vi "DigSeqLogic_On_Delay.vi"(8 "Time":dbl=-1.0, 9 "Delay":dbl=1.0, 11 "Input":bool) -> (1 "Remain":dbl, 3 "Output":bool)   [LabVIEW 2019, in "Trajectory_Library.lvlib"]
doc: "This VI implements a digital \"on delay\". When input is zero, output is zero. When output is true, input goes true after the designated time delay. Once the delay counter has started, the time delay value cannot be changed.\n\nInputs:\n - Input -- Boolean input value\n - Delay -- On delay time in seconds.\n - Time -- Continously counting system time, Seconds. If not wired the FPGA time will be used.\n\nOutputs:\n - Output -- Boolean output value with the on delay applied\n - Remain -- Time remaining for this value to be off in, seconds. Value will be 0 to Delay input value."
uses:
  Trajectory_Library.lvlib
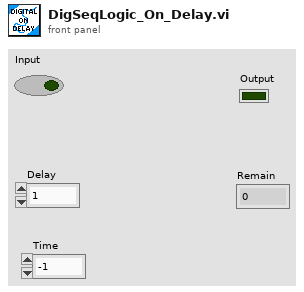
[diagram p1: front panel]
types:
  T1 = typedef "WPILib_Math.lvlib/TIMER.ctl" = cluster{"StartTime":dbl, "Accumulated TIme":dbl, "Running":bool, "semaphore":T2}
  T2 = typedef "Semaphore RefNum" = refnum<k1>
  T3 = typedef "Trajectory_Library.lvlib/TIMER.ctl" = cluster{"StartTime":dbl, "Accumulated TIme":dbl, "Running":bool, "semaphore":T2}
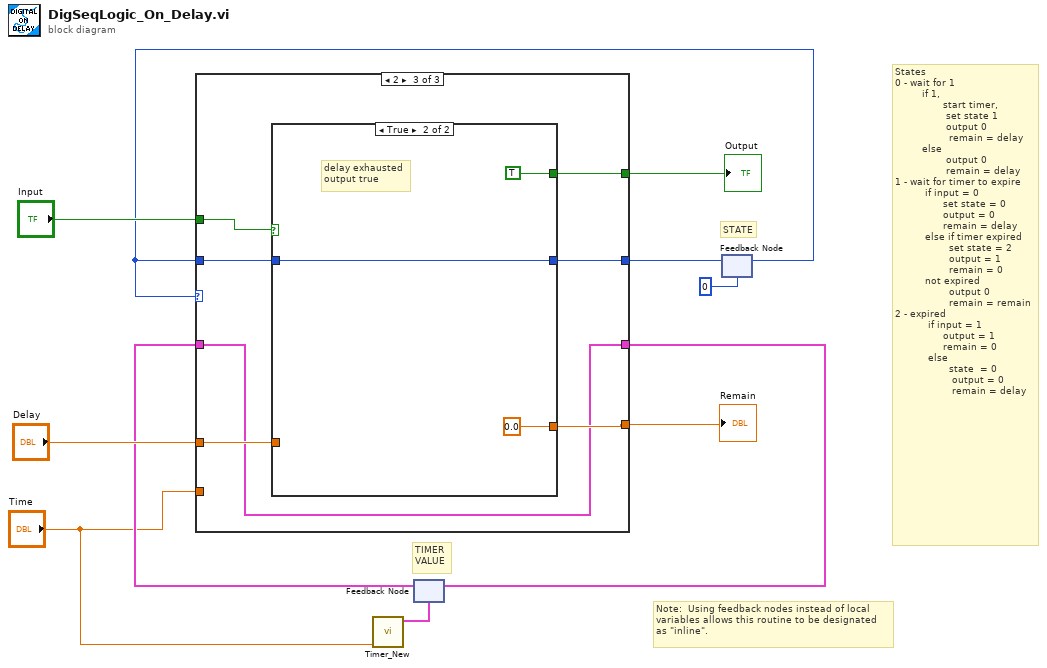
[diagram p0: block diagram]
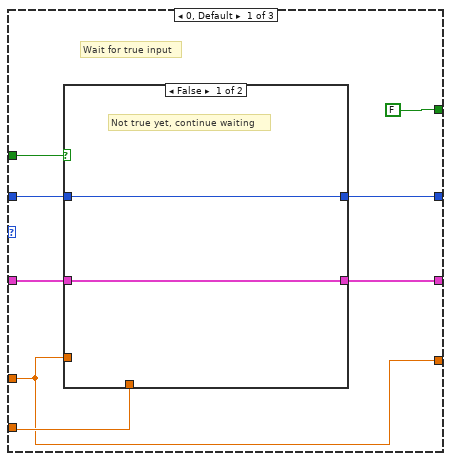
[diagram p2: hidden frame]
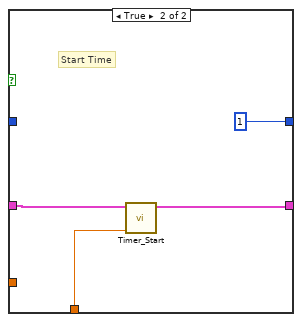
[diagram p3: hidden frame]
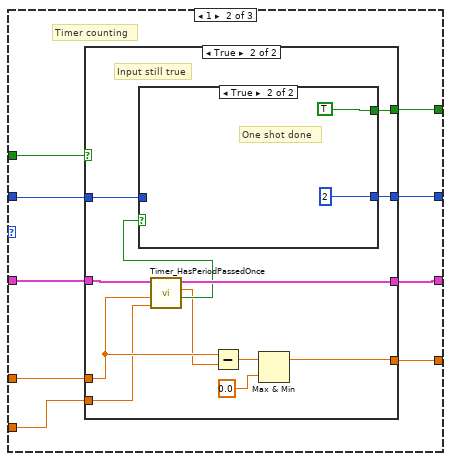
[diagram p4: hidden frame]
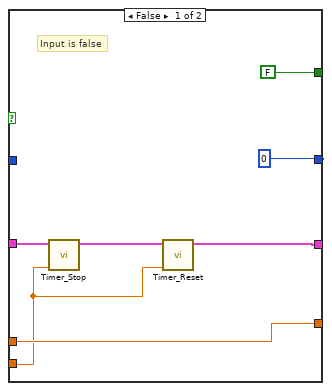
[diagram p5: hidden frame]
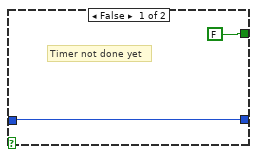
[diagram p6: hidden frame]
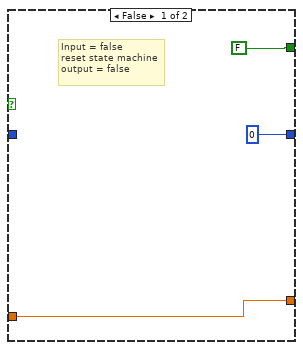
[diagram p7: hidden frame]
diagram:
  # "Note:  Using feedback nodes instead of local\nvariables allows this routine to be designated\nas \"inline\"."
  # "TIMER\nVALUE"
  # "STATE"
  # "States \n0 - wait for 1\n         if 1, \n                start timer, \n                 set state 1\n                 output 0\n                  remain = delay\n         else\n                 output 0\n                 remain = delay    \n1 - wait for timer to expire\n          if input = 0\n                set state = 0\n                output = 0\n                remain = delay\n          else if timer expired\n                  set state = 2\n                  output = 1\n                  remain = 0 \n          not expired\n                  output 0\n                  remain = remain\n2 - expired\n           if input = 1\n                output = 1\n                remain = 0\n           else\n                  state  = 0\n                   output = 0\n                   remain = delay"
  n1 = call "Timer_New.vi"("Pass_Through_Time"="Time") -> ("TIMER"=w4:T1)  [unwired: 10 in]
  n2 = feedback #1(w4) -> (w3:T3)
  n3 = feedback #2(0 ("State")) -> (w6:i32)
  n4 = case shown="2" w6 {
    tunnel: "Delay" -> [w16 w32 w62]
    tunnel: "Time" -> [w19 w30 _]
    tunnel: [FALSE ("Output") w34 w63] -> w10
    tunnel: [w16 w31 w61] -> w9
    tunnel: "Input" -> [w18 w33 w64]
    tunnel: [w15 w29 w60] -> w7
    tunnel: w6 -> [w14 w28 w59]
    tunnel: [w13 w26 w58] -> w2
    tunnel: w3 -> [w12 w27 w58]
    frame 0, Default {
      # "Wait for true input"
      n5 = case shown="False" w18 {
        tunnel: w19 -> [_ w22]
        tunnel: w16 -> [_ _]
        tunnel: [w21 1 ("State")] -> w15
        tunnel: w14 -> [w21 _]
        tunnel: [w20 w23] -> w13
        tunnel: w12 -> [w20 w24]
        frame False {
          # "Not true yet, continue waiting"
        }
        frame True {
          # "Start Time"
          n6 = call "Timer_Start.vi"("Pass_Through_Time"=w22, "in Timer"=w24) -> ("out Timer"=w23:T1)  [unwired: 9 in]
        }
      }
    }
    frame 1 {
      # "Timer counting"
      n7 = case shown="True" w33 {
        tunnel: [FALSE w53] -> w34
        tunnel: [w40 w43] -> w31
        tunnel: w32 -> [w40 w45]
        tunnel: w30 -> [w35 w42]
        tunnel: [0 ("State") w52] -> w29
        tunnel: w28 -> [_ w51]
        tunnel: w27 -> [w38 w50]
        tunnel: [w36 w49] -> w26
        frame False {
          # "Input is false"
          n8 = call "Timer_Stop.vi"("Pass_Through_Time"=w35, "in Timer"=w38) -> ("out Timer"=w37:T3)  [unwired: 9 in]
          n9 = call "Timer_Reset.vi"("Pass_Through_Time"=w35, "in TIMER"=w37) -> ("out TIMER"=w36:T3)  [unwired: 9 in]
        }
        frame True {
          # "Input still true"
          n10 = call "Timer_HasPeriodPassedOnce.vi"("Pass_Through_Time"=w42, "Period"=w45, "in Timer"=w50) -> ("Expired"=w48:bool, "CurrentTImer"=w44:dbl, "out Timer"=w49:T3)  [unwired: 6 in]
          n11 = case shown="True" w48 {
            tunnel: [FALSE TRUE] -> w53
            tunnel: [w54 2 ("State")] -> w52
            tunnel: w51 -> [w54 _]
            frame False {
              # "Timer not done yet"
            }
            frame True {
              # "One shot done"
            }
          }
          n12 = Subtract(x=w45, y=w44) -> (x-y=w46:dbl)
          n13 = Max & Min(x=w46, y=0.0) -> (max(x,y)=w43:dbl)  [unwired: 1 out]
        }
      }
    }
    frame 2 {
      n14 = case shown="True" w64 {
        tunnel: [FALSE TRUE] -> w63
        tunnel: w62 -> [w66 _]
        tunnel: [w66 0.0 ("Delay")] -> w61
        tunnel: [0 ("State") w68] -> w60
        tunnel: w59 -> [_ w68]
        frame False {
          # "Input = false\nreset state machine\noutput = false"
        }
        frame True {
          # "delay exhausted\noutput true"
        }
      }
    }
  }
  "Remain" <- w9
  "Output" <- w10
  n15 = feedback-in #1(w2) -> ()
  n16 = feedback-in #2(w7) -> ()
